vi "ConvertBoolToString.vi"(11 "Boolean":bool) -> (3 "String":string)   [LabVIEW 2013]
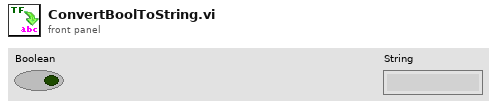
[diagram p1: front panel]
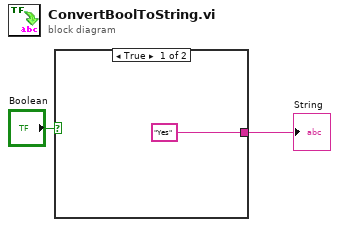
[diagram p0: block diagram]
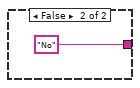
[diagram p2: hidden frame]
diagram:
  n1 = case shown="True" "Boolean" {
    tunnel: ["Yes" "No"] -> w1
    frame True {
    }
    frame False {
    }
  }
  "String" <- w1
